vi "Read Drag Timeout.vi"(8 "error in (no error)":errorcluster, 11 "QMenu Class in":refnum<class "QMenu Class.lvclass">) -> (0 "error out":errorcluster, 2 "Drag Timeout":i32, 3 "QMenu Class out":refnum<class "QMenu Class.lvclass">)   [LabVIEW 2020, in "QTab.lvlib" / "QMenu Class.lvclass"]
uses:
  QMenu Class.lvclass
  QMenu Class.lvclass/QMenu Class.ctl
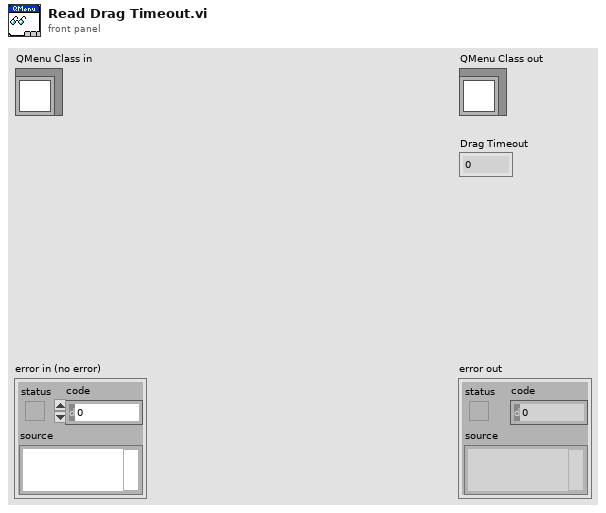
[diagram p1: front panel]
types:
  T1 = typedef "QTab.lvlib/QMenu Class.lvclass/Parameter.ctl" = cluster{"Close Timeout":i32, "Drag Timeout":i32}
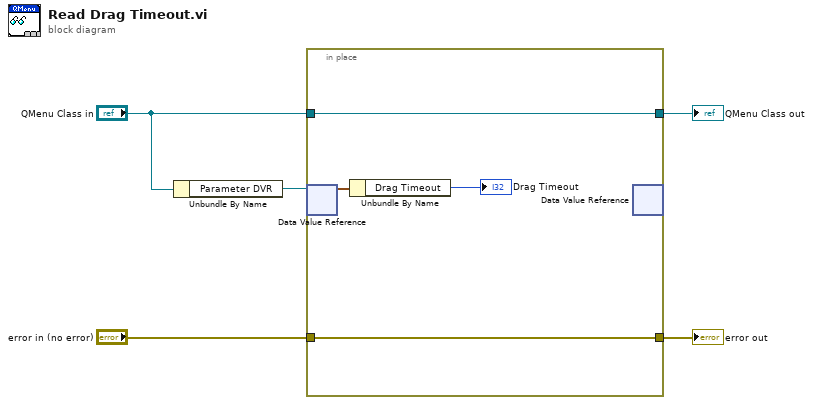
[diagram p0: block diagram]
diagram:
  n1 = Unbundle By Name("QMenu Class in") -> ("Parameter DVR"=w5:refnum<data-value>)
  n2 = in-place {
    in-place-border: "QMenu Class in" -> [w9]
    in-place-border: "error in (no error)" -> [w8]
    in-place-border: [w9] -> w2
    in-place-border: [w8] -> w1
    n3 = in-place-dvr #1(w5) -> (w7:T1)  [unwired: 1 out]
    n4 = Unbundle By Name(w7) -> ("Drag Timeout"=→"Drag Timeout":i32)
    n5 = in-place-dvr #1() -> ()  [unwired: 1 in, 2 out]
  }
  "error out" <- w1
  "QMenu Class out" <- w2
